vi "NewtonsPSM_Conf_LCR.vi"(0 "VISA session":refnum<visa-resource-name>, 1 "Condition (Auto Frequency)":u16(ring) items=["Auto Shunt", "Auto Frequency", "Manual"], 5 "Parameter (Auto)":u16(ring) items=["Auto", "Capacitance", "Inductance", "Impedance"], 7 "Model (Series)":u16(ring) items=["Series", "Parallel"], 9 "External Shunt (None)":u16(ring) items=["None", "Low", "Normal", "High", "Very High"], 11 "error in (no error)":errorcluster, 12 "Graph (Tan d / QF)":u16(ring)=1 items=["Single", "Tan d / QF", "Resistance"], 13 "Impedance Graph y Axis (Linear)":u16(ring) items=["Linear", "Log"]) -> (4 "dup VISA session":refnum<visa-resource-name>, 15 "error out":errorcluster)   [LabVIEW 2025, in "NewtonsPSM1735.lvlib"]
doc: "This VI set the LCR mode parameters to the PPA2530."
uses:
  NewtonsPSM1735.lvlib
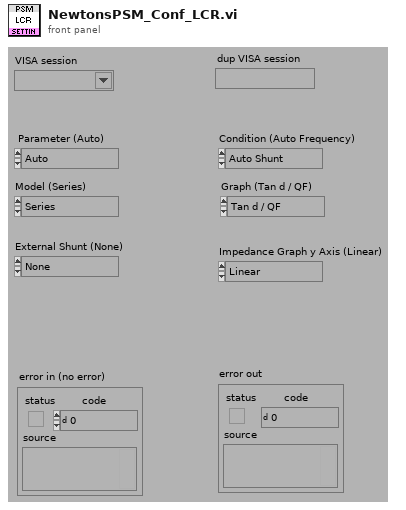
[diagram p1: front panel]
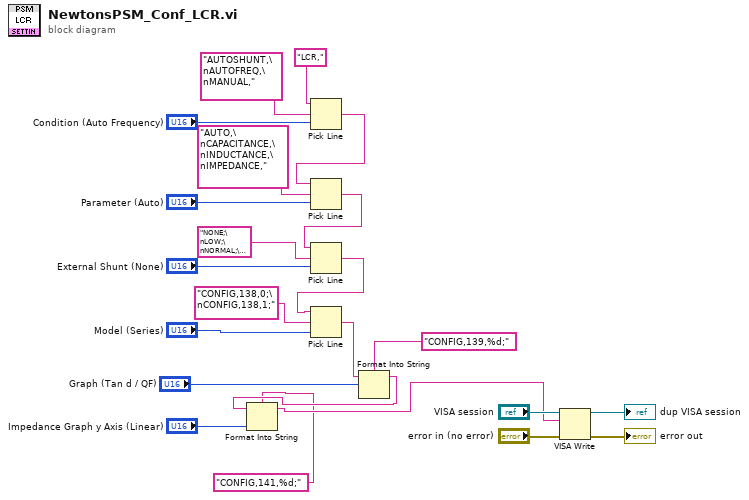
[diagram p0: block diagram]
diagram:
  n1 = Pick Line(string ("")="LCR,", multi-line string="AUTOSHUNT,\nAUTOFREQ,\nMANUAL,", line index="Condition (Auto Frequency)") -> (output string=w12:string)
  n2 = Pick Line(string ("")=w12, multi-line string="AUTO,\nCAPACITANCE,\nINDUCTANCE,\nIMPEDANCE,", line index="Parameter (Auto)") -> (output string=w8:string)
  n3 = Pick Line(string ("")=w8, multi-line string="NONE;\nLOW;\nNORMAL;\nHIGH;\nVHIGH", line index="External Shunt (None)") -> (output string=w6:string)
  n4 = Pick Line(string ("")=w6, multi-line string="CONFIG,138,0;\nCONFIG,138,1;", line index="Model (Series)") -> (output string=w15:string)
  n5 = Format Into String(format string="CONFIG,139,%d;", initial string=w15, "Graph (Tan d / QF)") -> (resulting string=w3:string)  [unwired: 1 in, 1 out]
  n6 = Format Into String(format string="CONFIG,141,%d;", initial string=w3, "Impedance Graph y Axis (Linear)") -> (resulting string=w2:string)  [unwired: 1 in, 1 out]
  n7 = VISA Write(VISA resource name="VISA session", write buffer=w2, error in (no error)="error in (no error)") -> (VISA resource name out=→"dup VISA session":refnum<visa-resource-name>, error out=→"error out":errorcluster)  [unwired: 1 out]
